vi "Start Iterations.vi"(8 "error in (no error)":errorcluster, 11 "Abstract Iterator Actor in":refnum<class "Abstract Iterator Actor.lvclass">) -> (0 "error out":errorcluster, 3 "Abstract Iterator Actor out":refnum<class "Abstract Iterator Actor.lvclass">)   [LabVIEW 2023, in "Iterator Actor.lvlib" / "Abstract Iterator Actor.lvclass"]
doc: "Starts the sequence of iterations."
uses:
  Abstract Iterator Actor.lvclass
  Abstract Iterator Actor.lvclass/Abstract Iterator Actor.ctl
  Abstract Iterator Actor Messages/Iterator Msg/Iterator Msg.lvclass
  <vilib>/LS Instruments AG/Async Methods Actor/Async Methods Actor/Async Methods Actor/Async Call Method.ctl
  Abstract Iterator Actor Messages/Acknowledge Itetations End Msg/Acknowledge Itetations End Msg.lvclass
  <vilib>/ActorFramework/Actor/Actor.lvclass/Actor.ctl
  <vilib>/ActorFramework/Message Enqueuer/Message Enqueuer.lvclass/Message Enqueuer.ctl
  <vilib>/LS Instruments AG/Async Methods Actor/Async Methods Actor/Async Methods Actor Messages/Async Message/Async Message.lvclass/Async Message.ctl
  <vilib>/LS Instruments AG/Async Methods Actor/Async Methods Actor/Async Methods Actor Messages/Async Message/Write Completion Notification Msg.vi
  <vilib>/LS Instruments AG/Async Methods Actor/Async Methods Actor/Async Methods Actor Messages/Async Message/Write Caller Enqueuer.vi
  <vilib>/ActorFramework/Message Enqueuer/Init from Existing Queue.vi
  <vilib>/ActorFramework/Message Enqueuer/Enqueue.vi
  <vilib>/LS Instruments AG/Async Methods Actor/Async Methods Actor/Async Methods Actor Messages/Async Message/Async Message.lvclass
  <vilib>/string/Create NI GUID.vi
  <vilib>/ActorFramework/Message Priority Queue/Priority Enqueue.vi
  <vilib>/ActorFramework/Message Enqueuer/Message Enqueuer.lvclass
  <vilib>/ActorFramework/Actor/Actor.lvclass
  <vilib>/LS Instruments AG/Async Methods Actor/Async Methods Actor/Async Methods Actor/Async Methods Actor.lvclass
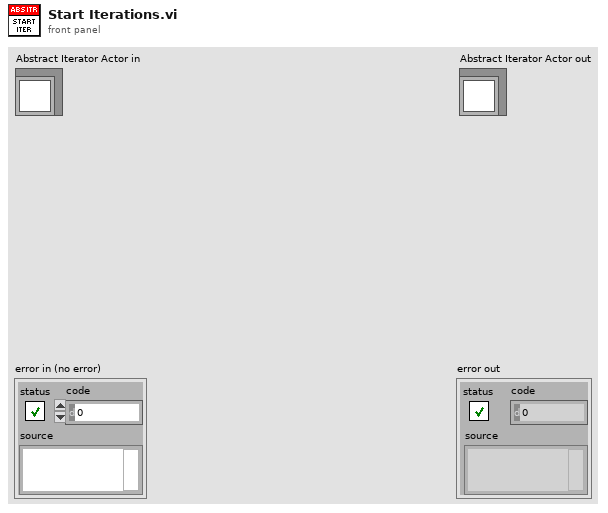
[diagram p1: front panel]
types:
  T1 = typedef "Async Methods Actor.lvlib/Async Methods Actor.lvclass/Async Call Method.ctl" = enum16{"Call and Collect", "Call and Forget"}
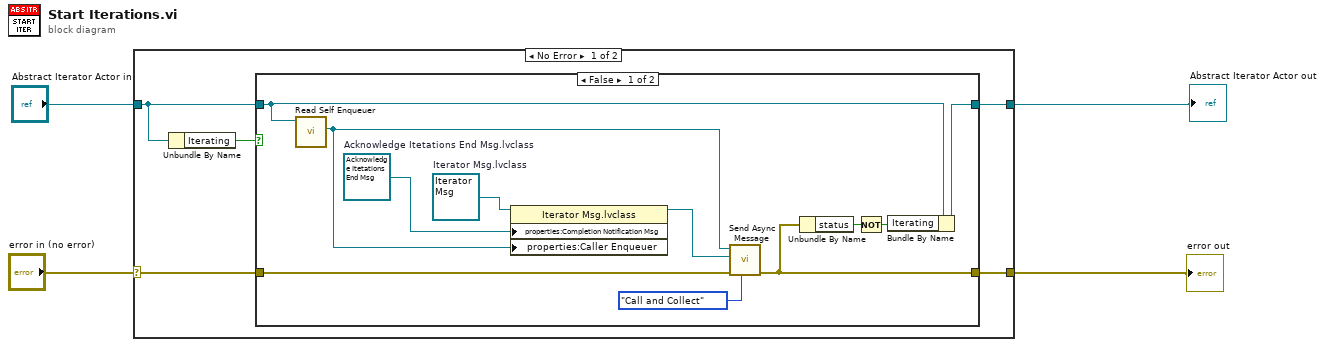
[diagram p0: block diagram]
diagram:
  n1 = case shown="No Error" "error in (no error)" {
    selector: "error in (no error)" -> [w9 w24]
    tunnel: [w8 w24] -> w3
    tunnel: [w7 w23] -> w1
    tunnel: "Abstract Iterator Actor in" -> [w6 w23]
    frame No Error {
      n2 = Unbundle By Name(w6) -> ("Iterating"=w5:bool)
      n3 = case shown="False" w5 {
        tunnel: w9 -> [w17 w21]
        tunnel: [w14 w21] -> w8
        tunnel: [w13 w22] -> w7
        tunnel: w6 -> [w10 w22]
        frame False {
          w15 = refnum<class "Acknowledge Itetations End Msg.lvclass"> refnum  # Acknowledge Itetations End Msg.lvclass
          w18 = refnum<class "Iterator Msg.lvclass"> refnum  # Iterator Msg.lvclass
          n4 = call <vilib>:"Read Self Enqueuer.vi"("Actor"=w10) -> ("Self Enqueuer"=w16:refnum<class "Message Enqueuer.lvclass">)  [unwired: 10 in]
          n5 = property class="Iterator Msg.lvclass"(reference=w18, "properties:Completion Notification Msg"=w15, "properties:Caller Enqueuer"=w16) -> (reference out=w19:refnum<class "Iterator Msg.lvclass">)  [unwired: 1 in, 1 out]
          n6 = call <vilib>:"Send Async Message.vi"("Async Call Method (Call and Collect)"=Async_Call_Method."Call and Collect" ("Async Call Method"), "error in (no error)"=w17, "Concrete Async Message"=w19, "Message Enqueuer"=w16) -> ("error out"=w14:errorcluster)  [unwired: 5 in, 2 out]
          n7 = Unbundle By Name(w14) -> ("status"=w12:bool)
          n8 = Not(x=w12) -> (.not. x?=w11:bool)
          n9 = Bundle By Name(cluster=w10, "Iterating"=w11) -> (w13:refnum<class "Abstract Iterator Actor.lvclass">)
        }
        frame True {
          # "#todo throw error"
        }
      }
    }
    frame Error {
    }
  }
  "error out" <- w3
  "Abstract Iterator Actor out" <- w1
